vi "PulseGeneratorSelect.vi"(0 "Serial port name":refnum<visa-resource-name>, 2 "start commands":string[](array[string]), 3 "stop commands":string[](array[string])) -> (6 "pulse buffer":T1, 8 "error out":errorcluster)   [LabVIEW 2014]
uses:
  <vilib>/Instr/_visa.llb/VISA Flush IO Buffer Mask.ctl
  <vilib>/Instr/_visa.llb/VISA Configure Serial Port (Instr).vi
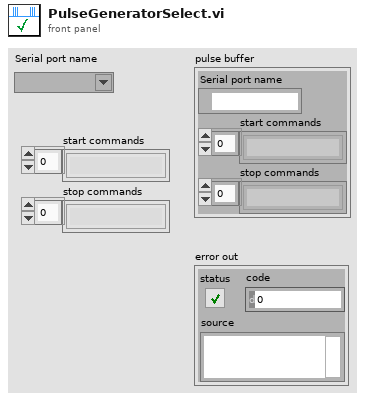
[diagram p1: front panel]
types:
  T1 = cluster{"Serial port name":refnum<visa-resource-name>, "start commands":string[], "stop commands":string[]}
  T2 = typedef "VISA Flush IO Buffer Mask.ctl" = u16
  T3 = cluster{"VISA resource name out":refnum<visa-resource-name>, "start commands":string[], "stop commands":string[]}
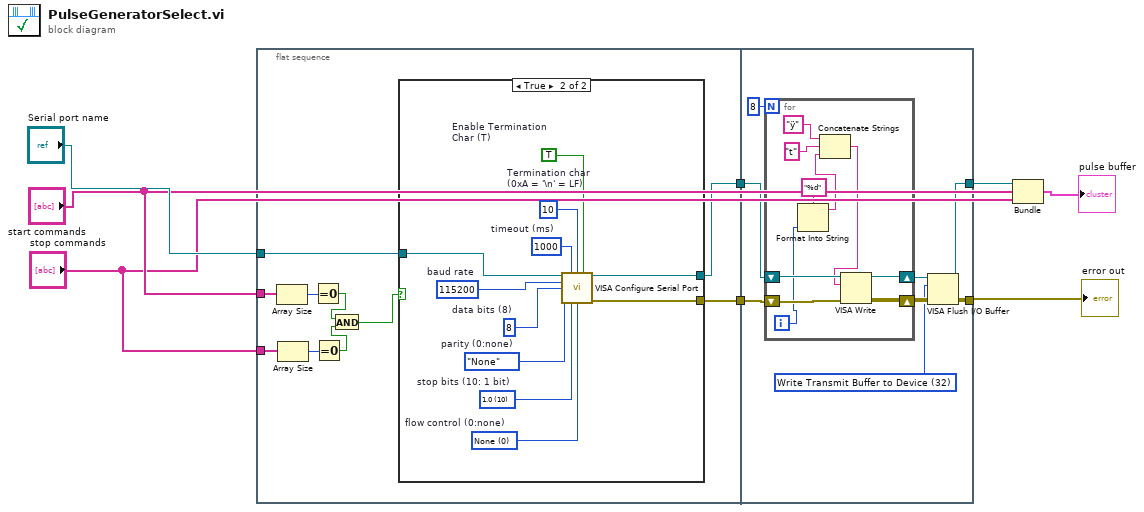
[diagram p0: block diagram]
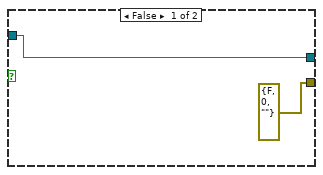
[diagram p2: hidden frame]
diagram:
  n1 = flat-sequence {
    tunnel: "Serial port name" -> [w9]
    tunnel: "start commands" -> [w14]
    tunnel: "stop commands" -> [w13]
    tunnel: [w12] -> w2
    tunnel: [w11] -> w1
    tunnel: [w34] -> w3
    tunnel: [w36] -> w4
    tunnel: w2 -> [w38]
    tunnel: w1 -> [w39]
    frame #0 {
      n2 = Array Size(array=w14) -> (size(s)=w18:i32)
      n3 = Array Size(array=w13) -> (size(s)=w17:i32)
      n4 = Equal To 0?(x=w18) -> (x = 0?=w15:bool)
      n5 = Equal To 0?(x=w17) -> (x = 0?=w16:bool)
      n6 = And(x=w15, y=w16) -> (x .and. y?=w10:bool)
      n7 = case shown="True" w10 {
        tunnel: [w19 w22] -> w12
        tunnel: [errorcluster {"status"=FALSE, "code"=0, "source"=""} ("error constant") w21] -> w11
        tunnel: w9 -> [w19 w23]
        frame False {
        }
        frame True {
          w24 = TRUE  # Enable Termination Char (T)
          w25 = u8 10  # Termination char (0xA = '\n' = LF)
          w26 = u16 0 items=["None", "XON/XOFF", "RTS/CTS", "XON/XOFF & RTS/CTS", "DTR/DSR", "XON/XOFF & DTR/DSR"]  # flow control (0:none)
          w27 = u16 10 items=["1.0"=10, "1.5"=15, "2.0"=20]  # stop bits (10: 1 bit)
          w28 = u32 1000  # timeout (ms)
          w29 = enum16{"None", "Odd", "Even", "Mark", "Space"}."None"  # parity (0:none)
          w30 = u16 8  # data bits (8)
          w31 = u32 115200  # baud rate
          n8 = call-poly "VISA Configure Serial Port"("VISA resource name"=w23, "timeout (10sec)"=w28, "termination char\n(0xA = '\\n' = LF)"=w25, "Enable Termination\nChar (T)"=w24, "baud rate (9600)"=w31, "data bits (8)"=w30, "parity (0:none)"=w29, "stop bits (10: 1 bit)"=w27, "flow control (0:none)"=w26) -> ("VISA resource name out"=w22:refnum<visa-resource-name>, "error out"=w21:errorcluster)  [unwired: 5 in]
        }
      }
    }
    frame #1 {
      w33 = T2 32 items=["Flush Receive Buffer"=16, "Write Transmit Buffer to Device"=32, "Flush Receive Buffer (No I/O)"=64, "Flush Transmit Buffer"=128] ("Mask")
      n9 = for {
        N: 8 -> [_]
        shift-right: [w43] -> w35
        shift-left: w39 -> [w49]
        shift-right: [w44] -> w37
        shift-left: w38 -> [w48]
        i -> [w40]
        n10 = Format Into String(format string="%d", w40) -> (resulting string=w41:string)  [unwired: 2 in, 1 out]
        n11 = Concatenate Strings("ÿ" ("string"), "t" ("string"), w41) -> (w47:string)
        n12 = VISA Write(VISA resource name=w48, write buffer=w47, error in (no error)=w49) -> (VISA resource name out=w44:refnum<visa-resource-name>, error out=w43:errorcluster)  [unwired: 1 out]
      }
      n13 = VISA Flush I/O Buffer(VISA resource name=w37, mask (16)=w33, error in (no error)=w35) -> (VISA resource name out=w36:refnum<visa-resource-name>, error out=w34:errorcluster)
    }
  }
  n14 = Bundle("VISA resource name out"=w4, "start commands"="start commands", "stop commands"="stop commands") -> (→"pulse buffer":T3)  [unwired: 1 in]
  "error out" <- w3
